vi "Connection Check.vi"(0 "Queue in":refnum<queue>, 1 "Producer State In":string, 2 "error in":errorcluster, 3 "error in (no error)":errorcluster, 4 "Connected":bool=TRUE, 5 "Receiving Data":bool=TRUE) -> (7 "Queue out":refnum<queue>, 8 "Producer State Out":string, 10 "error out":errorcluster)   [LabVIEW 2019]
uses:
  MessageFormat1.ctl
  <vilib>/Utility/error.llb/Error Cluster From Error Code.vi
  <vilib>/ErrorRing/Error Ring.xnode
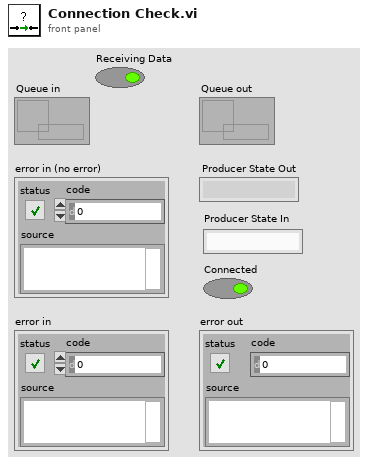
[diagram p1: front panel]
types:
  T1 = typedef "MessageFormat1.ctl" = cluster{"Consumer State":string, "RxData":string, "error constant":errorcluster, "Producer State ":string, "Numeric":dbl}
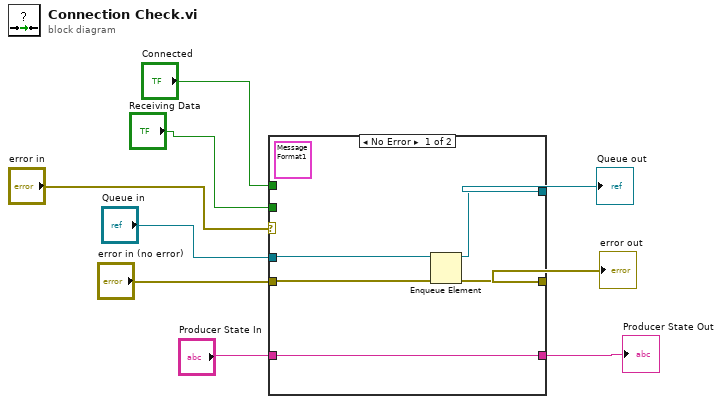
[diagram p0: block diagram]
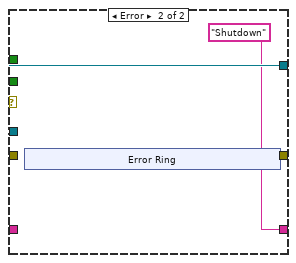
[diagram p2: hidden frame]
diagram:
  n1 = case shown="No Error" "error in" {
    tunnel: "error in (no error)" -> [w14 _]
    tunnel: "Queue in" -> [w13 w17]
    tunnel: [w12 w17] -> w6
    tunnel: [w11 w16] -> w8
    tunnel: [w10 "Shutdown" ("f")] -> w9
    tunnel: "Producer State In" -> [w10 _]
    tunnel: "Connected" -> [_ _]
    tunnel: "Receiving Data" -> [_ _]
    frame No Error {
      (unwired) T1 {"Consumer State"="Consumer State", "RxData"="Received Data", "error constant"={"status"=FALSE, "code"=0, "source"=""}, "Producer State "="Consumer State", "Numeric"=0.0} ("Queue Definition")
      n2 = Enqueue Element(queue=w13, error in (no error)=w14) -> (queue out=w12:refnum<queue>, error out=w11:errorcluster)  [unwired: 2 in, 1 out]
    }
    frame Error {
      n3 = xnode "Error Ring"() -> ("error out"=w16:errorcluster)
    }
  }
  "Producer State Out" <- w9
  "error out" <- w8
  "Queue out" <- w6
